vi "ReadAnyASCII.vi"(8 "error in (no error)":errorcluster, 11 "file path (dialog if empty)":path) -> (0 "error out":errorcluster, 1 "Header text":string, 2 "all rows":dbl[][](array[numeric]) format="%0.3f")   [LabVIEW 2021]
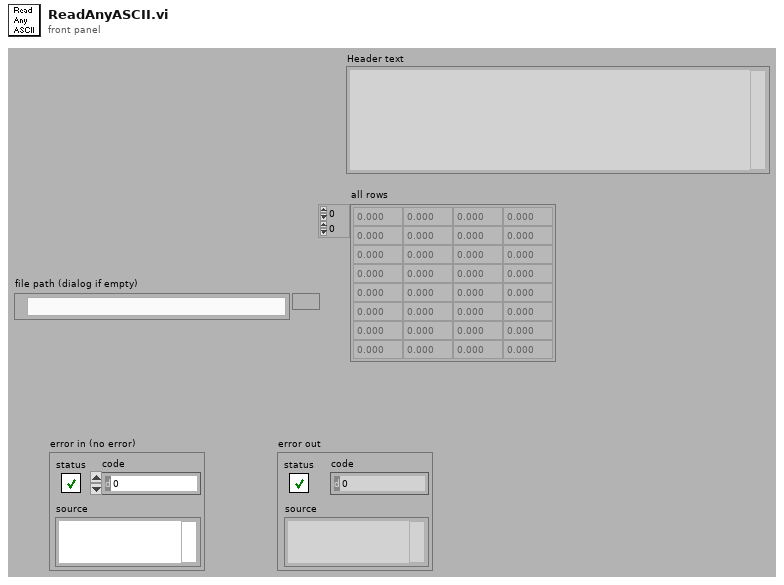
[diagram p1: front panel]
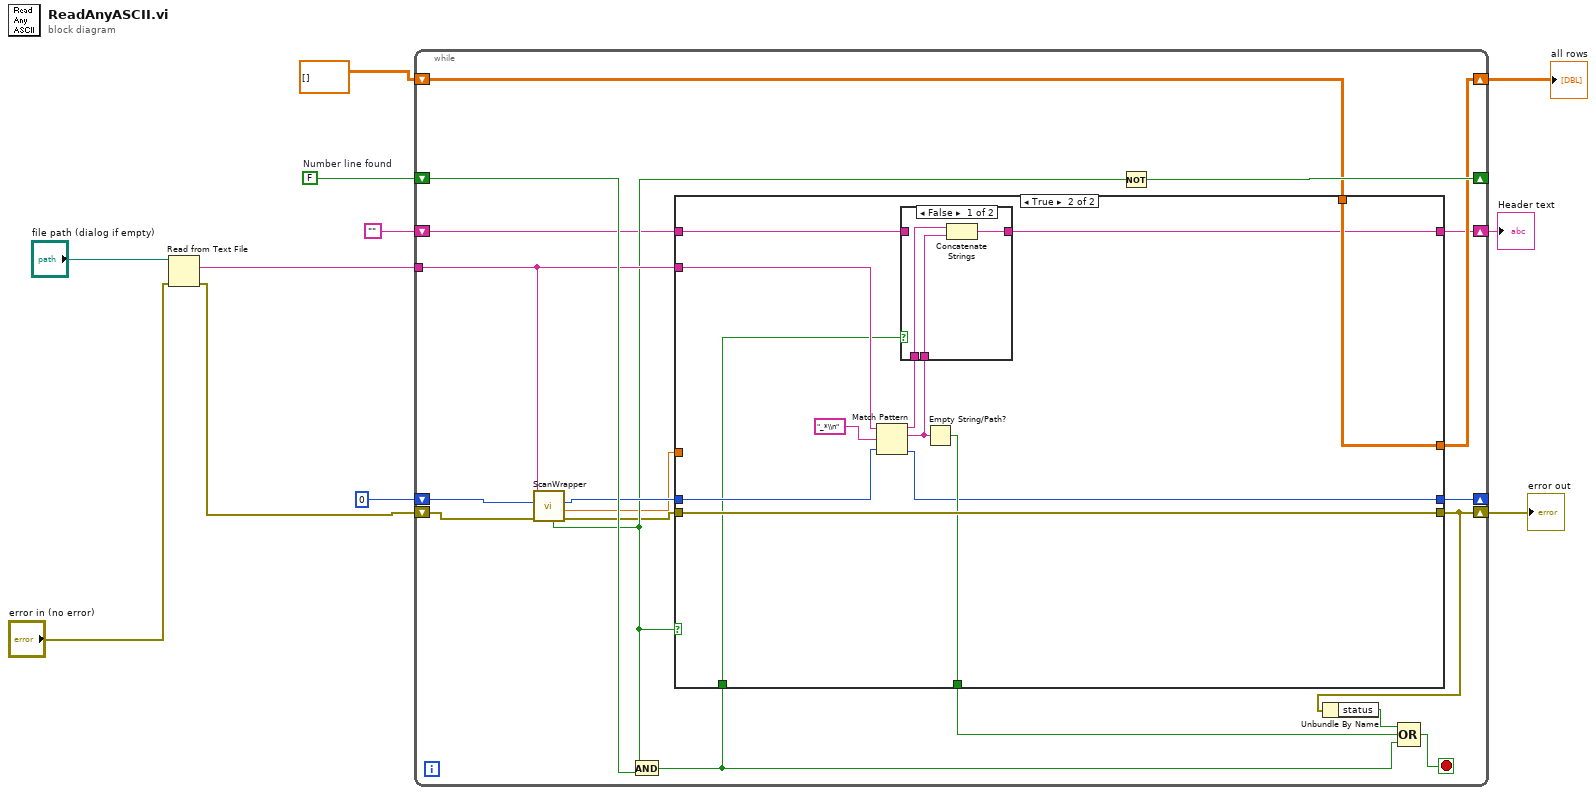
[diagram p0: block diagram]
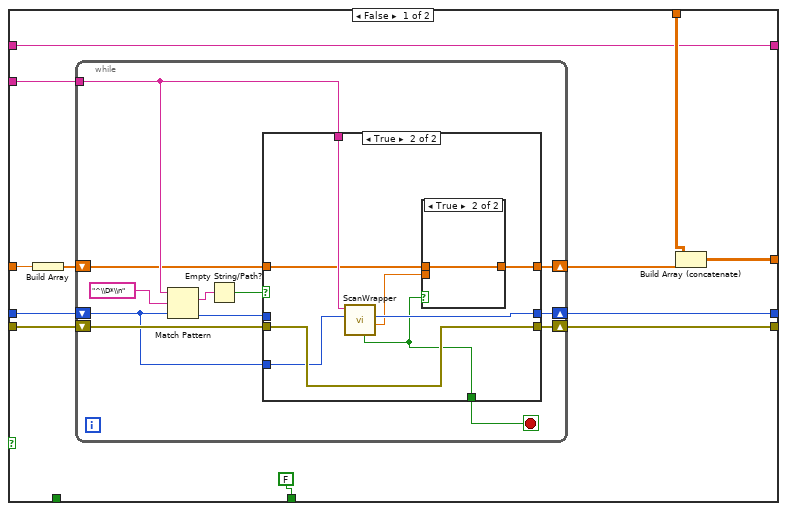
[diagram p2: hidden frame]
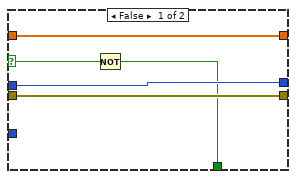
[diagram p3: hidden frame]
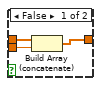
[diagram p4: hidden frame]
diagram:
  w10 = FALSE  # Number line found
  n1 = Read from Text File(file (use dialog)="file path (dialog if empty)", error in="error in (no error)") -> (text=w9:string, error out=w7:errorcluster)  [unwired: 4 out]
  n2 = while {
    shift-right: [w29] -> _
    shift-left: w10 -> [w28]
    tunnel: w9 -> [w25]
    shift-right: [w24] -> _
    shift-left: u32 0 -> [w30]
    shift-right: [w21] -> w5
    shift-left: w7 -> [w19]
    shift-right: [w22] -> w3
    shift-left: dbl[][] [] -> [w23]
    shift-right: [w12] -> w1
    shift-left: "" -> [w14]
    stop <- w27 stop-if-true
    n3 = call "ScanWrapper.vi"("error in (no error)"=w19, "initial scan location"=w30, "input string"=w25) -> ("error out"=w17:errorcluster, "output 1"=w18:dbl, "offset past scan"=w26:u32, "No number found"=w20:bool)  [unwired: 3 in, 2 out]
    n4 = And(x=w20, y=w28) -> (x .and. y?=w13:bool)
    n5 = case shown="True" w20 {
      tunnel: w17 -> [w42 w82]
      tunnel: [w41 w82] -> w21
      tunnel: w18 -> [w40 _]
      tunnel: w26 -> [w38 w79]
      tunnel: w25 -> [w37 w80]
      tunnel: [w36 w77] -> w24
      tunnel: w23 -> [w35 w83]
      tunnel: [w33 w83] -> w22
      tunnel: [FALSE w78] -> w15
      tunnel: w14 -> [w31 w76]
      tunnel: w13 -> [_ w75]
      tunnel: [w31 w72] -> w12
      frame False {
        n6 = Build Array(w40) -> (w39:dbl[])
        n7 = while {
          shift-right: [w54] -> w41
          shift-left: w42 -> [w53]
          shift-right: [w49] -> w34
          shift-left: w39 -> [w48]
          shift-right: [w47] -> w36
          shift-left: w38 -> [w43]
          tunnel: w37 -> [w50]
          stop <- w45 stop-if-true
          n8 = Match Pattern(string=w50, regular expression="^\\D*\\n", offset (0)=w43) -> (match substring=w51:string, offset past match=w44:i32)  [unwired: 2 out]
          n9 = Empty String/Path?(string/path=w51) -> (empty?=w46:bool)
          n10 = case shown="True" w46 {
            selector: w46 -> [w56 _]
            tunnel: [w57 w63] -> w54
            tunnel: w53 -> [w57 w63]
            tunnel: w44 -> [w59 _]
            tunnel: w50 -> [_ w67]
            tunnel: [w58 w66] -> w49
            tunnel: w48 -> [w58 w65]
            tunnel: [w59 w64] -> w47
            tunnel: [w55 w61] -> w45
            tunnel: w43 -> [_ w60]
            frame False {
              n11 = Not(x=w56) -> (.not. x?=w55:bool)
            }
            frame True {
              n12 = call "ScanWrapper.vi"("initial scan location"=w60, "input string"=w67) -> ("output 1"=w62:dbl, "offset past scan"=w64:u32, "No number found"=w61:bool)  [unwired: 3 in, 4 out]
              n13 = case shown="True" w61 {
                tunnel: [w68 w71] -> w66
                tunnel: w65 -> [w70 w71]
                tunnel: w62 -> [w69 _]
                frame False {
                  n14 = Build Array (concatenate)(w70, w69) -> (w68:dbl[])
                }
                frame True {
                }
              }
            }
          }
        }
        n15 = Build Array (concatenate)(w35, w34) -> (w33:dbl[][])
      }
      frame True {
        n16 = Match Pattern(string=w80, regular expression="_*\\n", offset (0)=w79) -> (before substring=w74:string, match substring=w73:string, offset past match=w77:i32)  [unwired: 1 out]
        n17 = case shown="False" w75 {
          tunnel: w76 -> [_ w87]
          tunnel: w74 -> [w86 _]
          tunnel: w73 -> [w85 _]
          tunnel: [w84 w87] -> w72
          frame False {
            n18 = Concatenate Strings(w86, w85) -> (w84:string)
          }
          frame True {
          }
        }
        n19 = Empty String/Path?(string/path=w73) -> (empty?=w78:bool)
      }
    }
    n20 = Not(x=w20) -> (.not. x?=w29:bool)
    n21 = Unbundle By Name(w21) -> ("status"=w16:bool)
    n22 = Compound Arithmetic op=OR(w16, w15, w13) -> (w27:bool)
  }
  "all rows" <- w3
  "error out" <- w5
  "Header text" <- w1
